vi "PumpValve3.vi"() -> ()   [LabVIEW 2015]
uses:
  PumpValve.ctl
  <vilib>/DAQmx/write.llb/DAQmx Write (Digital 1D Bool NChan 1Samp 1Line).vi
  <vilib>/DAQmx/miscellaneous.llb/DAQmx Fill In Error Info.vi
panel:
  in  "stop":bool
  out "Invalid fill%":bool
  out "Tank":u32(slide) scale=0.0..100.0
  in  "Drain %":u32
  in  "Fill %":u32
  in  "Drain":bool
  in  "Stop Program":bool
  in  "Fill":bool
  out "Green":i32
  out "Blue":i32
  out "Pump":i32
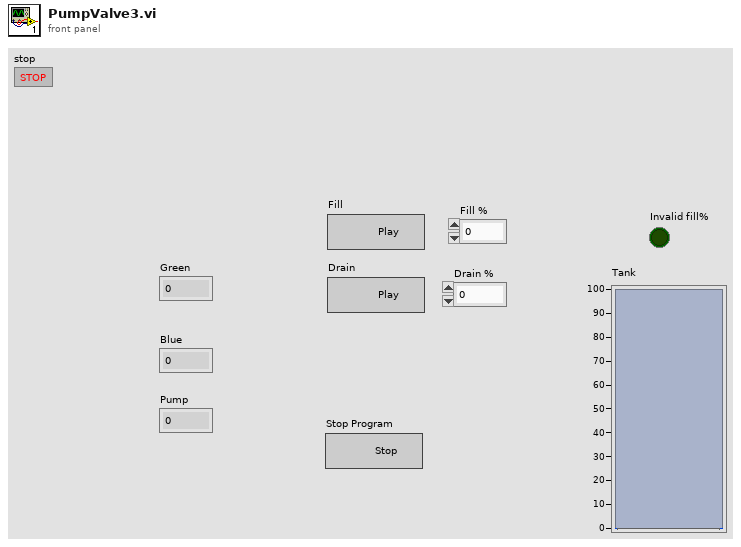
[diagram p1: front panel]
types:
  T1 = typedef "PumpValve.ctl" = enum16{"Initialize", "Idle", "Fill", "Drain", "Stop"}
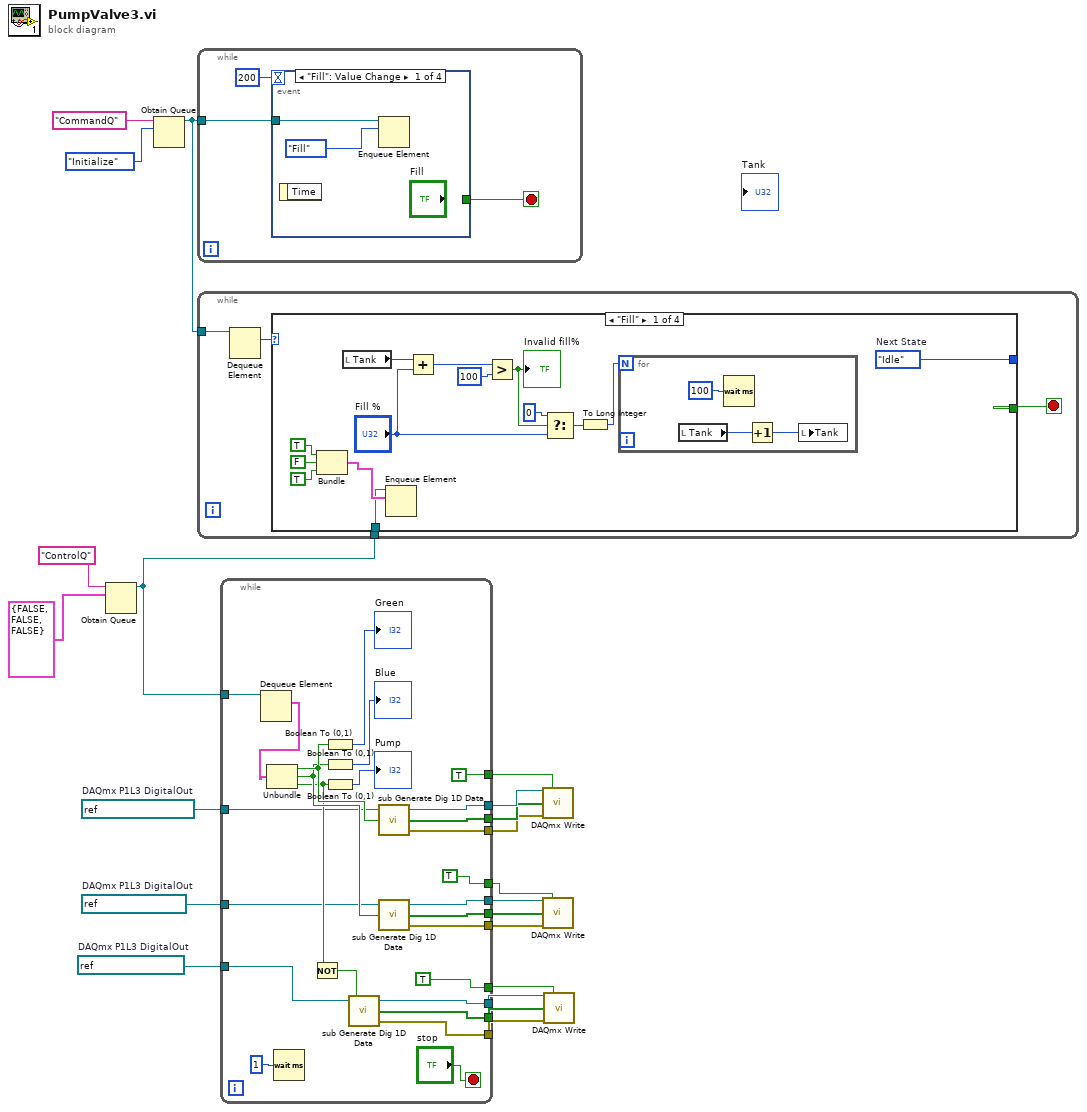
[diagram p0: block diagram]
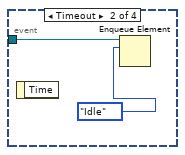
[diagram p2: hidden frame]
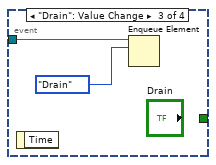
[diagram p3: hidden frame]
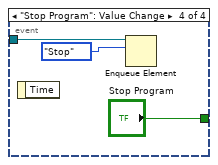
[diagram p4: hidden frame]
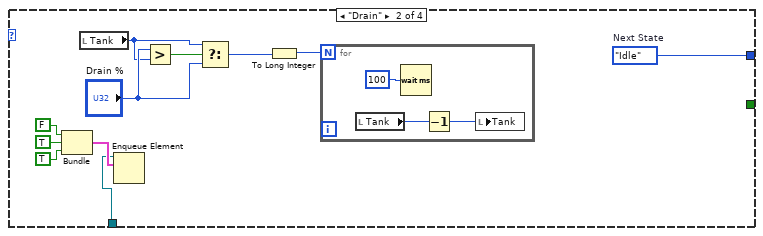
[diagram p5: hidden frame]
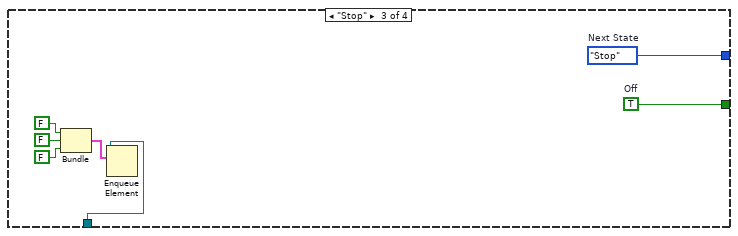
[diagram p6: hidden frame]
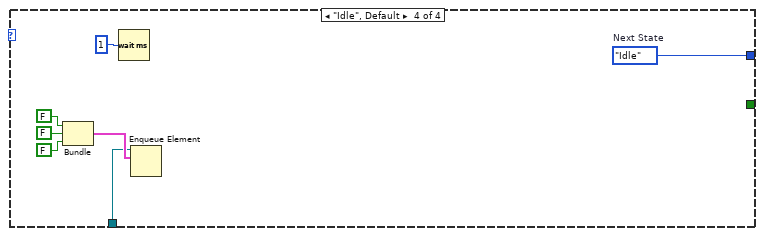
[diagram p7: hidden frame]
diagram:
  w19 = refnum<k21> "P0L0DigitalOut"  # DAQmx P1L3 DigitalOut
  w18 = refnum<k21> "DigitalOutBlue"  # DAQmx P1L3 DigitalOut
  w17 = refnum<k21> "DigitalOutGreen"  # DAQmx P1L3 DigitalOut
  n1 = Obtain Queue(name (unnamed)="ControlQ", element data type=cluster{bool, bool, bool} {FALSE, FALSE, FALSE}) -> (queue out=w2:refnum<queue>)  [unwired: 3 in, 2 out]
  n2 = Obtain Queue(name (unnamed)="CommandQ", element data type=PumpValve."Initialize" ("States")) -> (queue out=w20:refnum<queue>)  [unwired: 3 in, 2 out]
  n3 = while {
    tunnel: w20 -> [w22]
    stop <- w23 stop-if-true
    n4 = event shown="[0] \"Fill\": Value Change" {
      selector: _ -> [_ _ _ _]
      dyn-events: _ -> [_ _ _ _]
      timeout: 200 -> [_ _ _ _]
      tunnel: [_ _ _ "Stop Program"] -> w23
      tunnel: w22 -> [w26 w28 w30 w33]
      event "Fill": Value Change {
        n5 = event-data() -> ()  [unwired: 1 in, 1 out]
        n6 = Enqueue Element(queue=w26, element=PumpValve."Fill" ("States")) -> ()  [unwired: 2 in, 3 out]
      }
      event Timeout {
        n7 = event-data() -> ()  [unwired: 1 in, 1 out]
        n8 = Enqueue Element(queue=w28, element=PumpValve."Idle" ("States")) -> ()  [unwired: 2 in, 3 out]
      }
      event "Drain": Value Change {
        n9 = event-data() -> ()  [unwired: 1 in, 1 out]
        n10 = Enqueue Element(queue=w30, element=PumpValve."Drain" ("States")) -> ()  [unwired: 2 in, 3 out]
      }
      event "Stop Program": Value Change {
        n11 = event-data() -> ()  [unwired: 1 in, 1 out]
        n12 = Enqueue Element(queue=w33, element=PumpValve."Stop" ("States")) -> ()  [unwired: 2 in, 3 out]
      }
    }
  }
  n13 = while {
    tunnel: w20 -> [w37]
    tunnel: w2 -> [w34]
    stop <- w36 stop-if-true
    n14 = Dequeue Element(queue=w37) -> (element=w35:T1)  [unwired: 2 in, 3 out]
    n15 = case shown="\"Fill\"" w35 {
      tunnel: [w51 w65 w75 w82] -> _
      tunnel: [_ _ w74 _] -> w36
      tunnel: w34 -> [w38 w55 w69 w76]
      frame "Fill" {
        w51 = PumpValve."Idle"  # Next State
        n16 = Bundle(TRUE, FALSE, TRUE) -> (w39:cluster{bool, bool, bool})  [unwired: 1 in]
        n17 = local read "Tank"() -> (w50:u32)
        n18 = Enqueue Element(queue=w38, element=w39) -> ()  [unwired: 2 in, 3 out]
        n19 = Add(x=w50, y="Fill %") -> (x+y=w48:u32)
        n20 = Greater?(x=w48, y=u32 100) -> (0:w45:bool)
        "Invalid fill%" <- w45
        n21 = Select(t=u32 0, s=w45, f="Fill %") -> (s? t:f=w44:u32)
        n22 = To Long Integer(number=w44) -> (32bit integer=w43:i32)
        n23 = for {
          N: w43 -> [_]
          n24 = local read "Tank"() -> (w54:u32)
          n25 = Wait (ms)(milliseconds to wait=u32 100 ("y")) -> ()  [unwired: 1 out]
          n26 = Increment(x=w54) -> (x+1=w53:u32)
          n27 = local write "Tank"(w53) -> ()
        }
      }
      frame "Drain" {
        w65 = PumpValve."Idle"  # Next State
        n28 = Bundle(FALSE, TRUE, TRUE) -> (w56:cluster{bool, bool, bool})  [unwired: 1 in]
        n29 = local read "Tank"() -> (w61:u32)
        n30 = Enqueue Element(queue=w55, element=w56) -> ()  [unwired: 2 in, 3 out]
        n31 = Greater?(x="Drain %", y=w61) -> (0:w64:bool)
        n32 = Select(t=w61, s=w64, f="Drain %") -> (s? t:f=w63:u32)
        n33 = To Long Integer(number=w63) -> (32bit integer=w60:i32)
        n34 = for {
          N: w60 -> [_]
          n35 = local read "Tank"() -> (w67:u32)
          n36 = Wait (ms)(milliseconds to wait=u32 100) -> ()  [unwired: 1 out]
          n37 = Decrement(x=w67) -> (x-1=w68:u32)
          n38 = local write "Tank"(w68) -> ()
        }
      }
      frame "Stop" {
        w74 = TRUE  # Off
        w75 = PumpValve."Stop"  # Next State
        n39 = Bundle(FALSE, FALSE, FALSE) -> (w70:cluster{bool, bool, bool})  [unwired: 1 in]
        n40 = Enqueue Element(queue=w69, element=w70) -> ()  [unwired: 2 in, 3 out]
      }
      frame "Idle", Default {
        w82 = PumpValve."Idle"  # Next State
        n41 = Bundle(FALSE, FALSE, FALSE) -> (w77:cluster{bool, bool, bool})  [unwired: 1 in]
        n42 = Wait (ms)(milliseconds to wait=u32 1) -> ()  [unwired: 1 out]
        n43 = Enqueue Element(queue=w76, element=w77) -> ()  [unwired: 2 in, 3 out]
      }
    }
  }
  n44 = while {
    tunnel: w2 -> [w84]
    tunnel: w19 -> [w101]
    tunnel: w18 -> [w100]
    tunnel: w17 -> [w99]
    tunnel: [TRUE] -> w16
    tunnel: [w97] -> w15
    tunnel: [w96] -> w14
    tunnel: [w95] -> w13
    tunnel: [TRUE] -> w12
    tunnel: [w93] -> w11
    tunnel: [w92] -> w10
    tunnel: [w91] -> w9
    tunnel: [TRUE] -> w8
    tunnel: [w89] -> w7
    tunnel: [w88] -> w6
    tunnel: [w87] -> w5
    stop <- "stop" stop-if-true
    n45 = Dequeue Element(queue=w84) -> (element=w83:cluster{bool, bool, bool})  [unwired: 2 in, 3 out]
    n46 = Unbundle(w83) -> (w104:bool, w103:bool, w102:bool)
    n47 = Wait (ms)(milliseconds to wait=u32 1) -> ()  [unwired: 1 out]
    n48 = Not(x=w102) -> (.not. x?=w107:bool)
    n49 = Boolean To (0,1)(Boolean=w104) -> (0, 1=→"Green":i16)
    n50 = Boolean To (0,1)(Boolean=w103) -> (0, 1=→"Blue":i16)
    n51 = Boolean To (0,1)(Boolean=w102) -> (0, 1=→"Pump":i16)
    n52 = call <vilib>:"sub Generate Dig 1D Data.vi"("initial value"=w107, "task in"=w101) -> ("error out"=w87:errorcluster, "Data"=w88:bool[], "task out"=w89:refnum<k21>)  [unwired: 1 in]
    n53 = call <vilib>:"sub Generate Dig 1D Data.vi"("initial value"=w104, "task in"=w99) -> ("error out"=w95:errorcluster, "Data"=w96:bool[], "task out"=w97:refnum<k21>)  [unwired: 1 in]
    n54 = call <vilib>:"sub Generate Dig 1D Data.vi"("initial value"=w103, "task in"=w100) -> ("error out"=w91:errorcluster, "Data"=w92:bool[], "task out"=w93:refnum<k21>)  [unwired: 1 in]
  }
  n55 = call-poly <vilib>:"DAQmx Write.vi"("task/channels in"=w15, "auto start"=w16, "data"=w14, "error in"=w13) -> ()  [unwired: 9 in, 3 out]
  n56 = call-poly <vilib>:"DAQmx Write.vi"("task/channels in"=w11, "auto start"=w12, "data"=w10, "error in"=w9) -> ()  [unwired: 9 in, 3 out]
  n57 = call-poly <vilib>:"DAQmx Write.vi"("task/channels in"=w7, "auto start"=w8, "data"=w6, "error in"=w5) -> ()  [unwired: 9 in, 3 out]
